vi "Broadcast_UDP_message.vi"(5 "message":string, 6 "error in":errorcluster, 8 "port (60434)":u16=60434, 9 "muliticast address":string="236.6.6.8") -> (0 "error out":errorcluster, 4 "responses":T1[](array[typedef]))   [LabVIEW 2014, in "Autodetect.lvlib"]
doc: "Broadcasts a message to the default multicast port for the devices.\n\nMulticast address = 236.6.6.8\nPort = 60434\n\nDefault message is *IDN? to return the hostname"
uses:
  Autodetect.lvlib
  TypeDefs/UDP_Response_TD.ctl
  <vilib>/Utility/tcp.llb/UDP Multicast Read-Write Open.vi
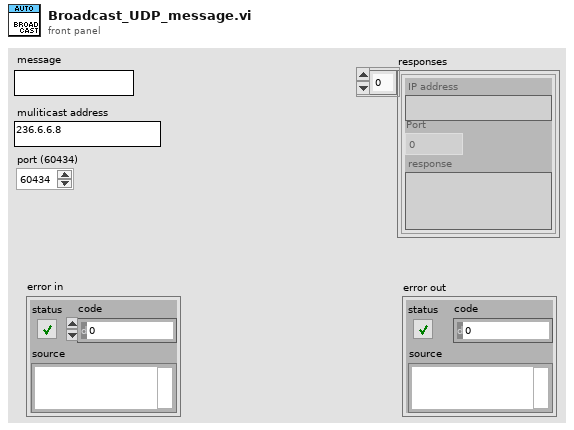
[diagram p1: front panel]
types:
  T1 = typedef "Autodetect.lvlib/UDP_Response_TD.ctl" = cluster{"IP address":string, "Port":u16, "response":string}
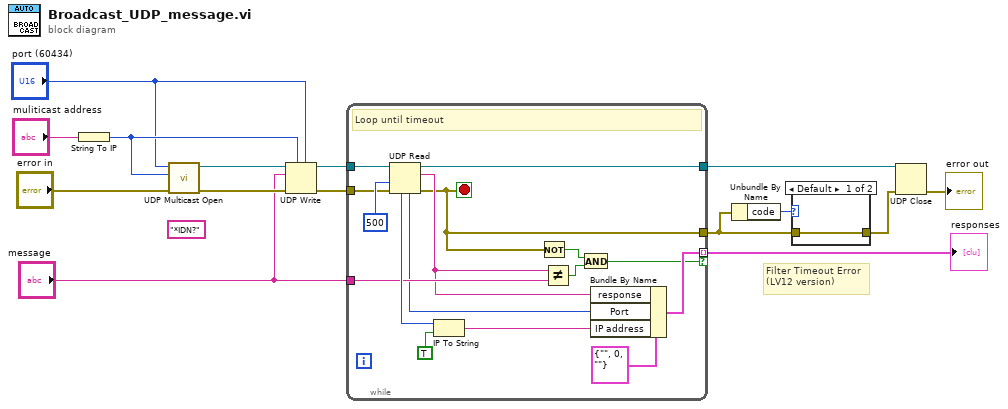
[diagram p0: block diagram]
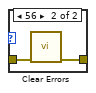
[diagram p2: hidden frame]
diagram:
  (unwired) "*IDN?" ("data in")
  # "Filter Timeout Error\n(LV12 version)"
  n1 = String To IP(1:"muliticast address") -> (0:w7:u32)
  n2 = call-poly <vilib>:"UDP Multicast Open.vi"("error in (no error)"="error in", "multicast addr"=w7, "port"="port (60434)") -> ("error out"=w13:errorcluster, "connection ID"=w14:refnum<k16>)  [unwired: 6 in, 1 out]
  n3 = UDP Write(address=w7, port or service name="port (60434)", connection ID=w14, data in="message", 8:w13) -> (error out=w10:errorcluster, 3:w11:refnum<k16>)  [unwired: 1 in]
  n4 = while {
    tunnel: w11 -> [w30]
    tunnel: w10 -> [w29]
    tunnel: [w19] -> w2
    tunnel: [w28] -> w9
    tunnel: [w23] -> w5 mode=indexing if=w16
    tunnel: "message" -> [w25]
    stop <- w19 stop-if-true
    # "Loop until timeout"
    n5 = UDP Read(connection ID=w30, timeout ms (25000)=500, 8:w29) -> (data out=w20:string, error out=w19:errorcluster, 3:w28:refnum<k16>, 4:w21:u16, 6:w26:u32)  [unwired: 1 out]
    n6 = IP To String(1:TRUE ("dot notation? (F)"), 2:w26) -> (0:w22:string)
    n7 = Not(x=w19) -> (.not. x?=w17:bool)
    n8 = Not Equal?(x=w20, y=w25) -> (x != y?=w18:bool)
    n9 = And(x=w17, y=w18) -> (x .and. y?=w16:bool)
    n10 = Bundle By Name(cluster=T1 {"IP address"="", "Port"=0, "response"=""}, "response"=w20, "Port"=w21, "IP address"=w22) -> (w23:T1)
  }
  "responses" <- w5
  n11 = Unbundle By Name(w2) -> ("code"=w1:i32)
  n12 = case shown="Default" w1 {
    tunnel: [w32 w34] -> w8
    tunnel: w2 -> [w32 w33]
    frame Default {
    }
    frame 56 {
      n13 = call <vilib>:"Clear Errors.vi"("error in (no error)"=w33) -> ("error out"=w34:errorcluster)  [unwired: 5 in, 1 out]
    }
  }
  n14 = UDP Close(connection ID=w9, 8:w8) -> (error out=→"error out":errorcluster)  [unwired: 1 out]
